vi "char_send.vi"(9 "Char to send":string="g", 10 "Input buffer size":u32=16384, 11 "USB Interface Name":refnum<visa-resource-name>="COM3") -> ()   [LabVIEW 2012]
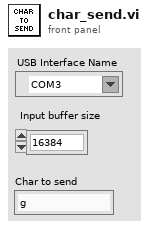
[diagram p1: front panel]
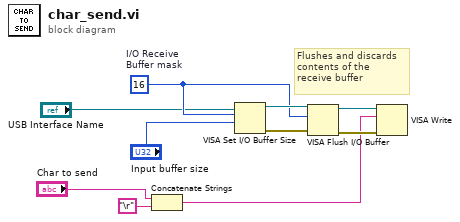
[diagram p0: block diagram]
diagram:
  w6 = u16 16  # I/O Receive Buffer mask
  # "Flushes and discards \ncontents of the \nreceive buffer"
  n1 = Concatenate Strings("Char to send", "\r") -> (w1:string)
  n2 = VISA Set I/O Buffer Size(VISA resource name="USB Interface Name", mask (16)=w6, size (4096)="Input buffer size") -> (VISA resource name out=w8:refnum<visa-resource-name>, error out=w7:errorcluster)  [unwired: 1 in]
  n3 = VISA Flush I/O Buffer(VISA resource name=w8, mask (16)=w6, error in (no error)=w7) -> (VISA resource name out=w10:refnum<visa-resource-name>, error out=w9:errorcluster)
  n4 = VISA Write(VISA resource name=w10, write buffer=w1, error in (no error)=w9) -> ()  [unwired: 3 out]
